vi "message.to.str.vi"(11 "OrderBook.Command[]":T1[](array[typedef])) -> (3 "Orderbook.Command[str]":string[](array[string]))   [LabVIEW 2020]
uses:
  Market.Data.Common/fpga/orderbook.command.ctl
  Market.Data.Common/fpga/orderbook.command.type.ctl
  Market.Data.Common/fpga/fpganow.common.fpga.lvlib
panel:
  out "orderId":u64
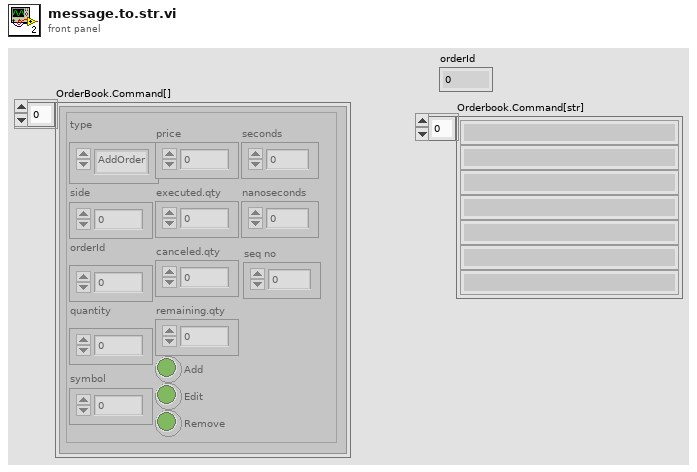
[diagram p1: front panel]
types:
  T1 = typedef "fpganow.common.fpga.lvlib/orderbook.command.ctl" = cluster{"type":T2, "side":u8, "orderId ":u64, "quantity":u32, "symbol":u64, "price":u64, "executed.qty":u32, "canceled.qty":u32, "remaining.qty":u32, "seconds":u64, "nanoseconds":u64, "Add":bool, "Edit":bool, "Remove":bool, "seq no":u32}
  T2 = typedef "fpganow.common.fpga.lvlib/orderbook.command.type.ctl" = enum8{"Time", "AddOrder", "OrderExecuted", "OrderExecutedAtPrice", "ReduceSize", "ModifyOrder", "DeleteOrder", "Get.Everything", "Get.All.Orders", "Get.Top"}
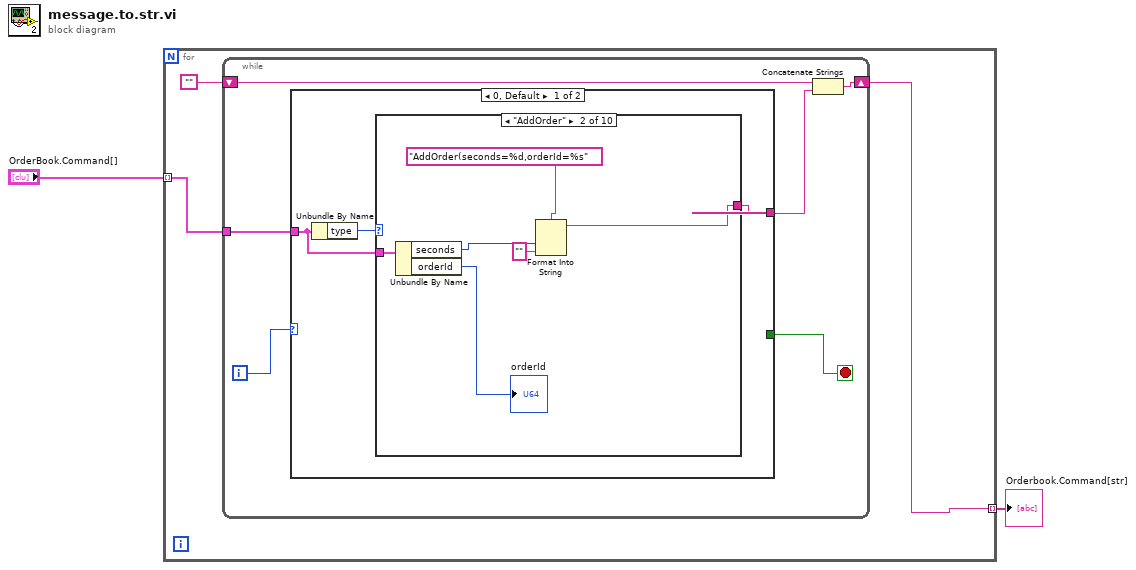
[diagram p0: block diagram]
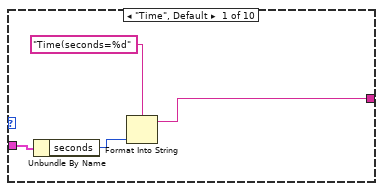
[diagram p2: hidden frame]
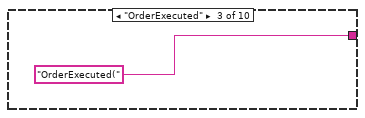
[diagram p3: hidden frame]
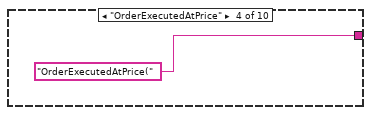
[diagram p4: hidden frame]
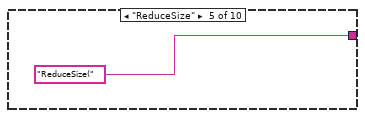
[diagram p5: hidden frame]
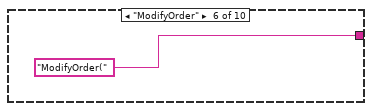
[diagram p6: hidden frame]
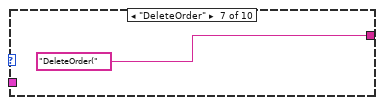
[diagram p7: hidden frame]
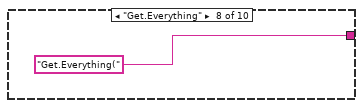
[diagram p8: hidden frame]
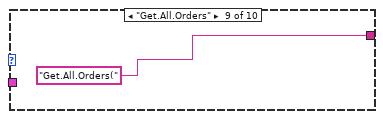
[diagram p9: hidden frame]
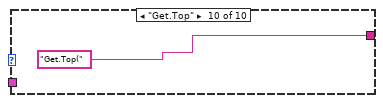
[diagram p10: hidden frame]
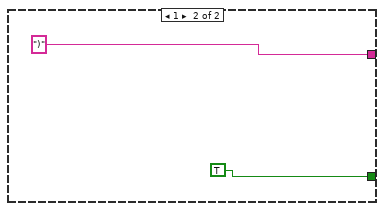
[diagram p11: hidden frame]
diagram:
  n1 = for {
    tunnel: "OrderBook.Command[]" -> [w3] mode=indexing
    tunnel: [w4] -> w1 mode=indexing
    n2 = while {
      shift-right: [w11] -> w4
      shift-left: "" -> [w8]
      tunnel: w3 -> [w6]
      i -> [w10]
      stop <- w9 stop-if-true
      n3 = case shown="0, Default" w10 {
        tunnel: [_ TRUE] -> w9
        tunnel: [w14 ")"] -> w7
        tunnel: w6 -> [w12 _]
        frame 0, Default {
          n4 = Unbundle By Name(w12) -> ("type"=w13:T2)
          n5 = case shown="\"AddOrder\"" w13 {
            tunnel: [w15 w21 "OrderExecuted(" "OrderExecutedAtPrice(" "ReduceSize(" "ModifyOrder(" "DeleteOrder(" "Get.Everything(" "Get.All.Orders(" "Get.Top("] -> w14
            tunnel: w12 -> [w18 w24 _ _ _ _ _ _ _ _]
            frame "Time", Default {
              n6 = Unbundle By Name(w18) -> ("seconds"=w17:u64)
              n7 = Format Into String(format string="Time(seconds=%d", w17) -> (resulting string=w15:string)  [unwired: 2 in, 1 out]
            }
            frame "AddOrder" {
              n8 = Unbundle By Name(w24) -> ("seconds"=w23:u64, "orderId"=→"orderId":u64)
              n9 = Format Into String(format string="AddOrder(seconds=%d,orderId=%s", w23, "" ("input 2")) -> (resulting string=w21:string)  [unwired: 2 in, 1 out]
            }
            frame "OrderExecuted" {
            }
            frame "OrderExecutedAtPrice" {
            }
            frame "ReduceSize" {
            }
            frame "ModifyOrder" {
            }
            frame "DeleteOrder" {
            }
            frame "Get.Everything" {
            }
            frame "Get.All.Orders" {
            }
            frame "Get.Top" {
            }
          }
        }
        frame 1 {
        }
      }
      n10 = Concatenate Strings(w8, w7) -> (w11:string)
    }
  }
  "Orderbook.Command[str]" <- w1
